vi "数据收集.vi"(8 "error in (no error)":errorcluster caption="错误输入（无错误）", 9 "DB5000.X":T1, 10 "Value":dbl format="%_3g", 11 "数组in":dbl[][](array[numeric])) -> (0 "error out":errorcluster caption="错误输出", 1 "添加的数组":dbl[](array[numeric]), 2 "连接的字符串":string, 3 "数组out":dbl[][](array[numeric]))   [LabVIEW 2017]
uses:
  <vilib>/Utility/file.llb/Write Delimited Spreadsheet (DBL).vi
panel:
  out "元素":bool
  out "F-格式字符串":string[](array[string])
  out "添加的数组 19":dbl[](array[numeric])
  out "MAX位置2":dbl format="%#_3g"
  out "添加的数组 20":dbl[](array[numeric])
  out "MAX位置1":dbl format="%#_3g"
  out "添加的数组 17":dbl[](array[numeric])
  out "MAX位置3":dbl format="%#_3g"
  out "添加的数组 18":dbl[](array[numeric])
  out "MAX位置18":dbl format="%#_3g"
  out "添加的数组 21":dbl[](array[numeric])
  out "MAX位置19":dbl format="%#_3g"
  out "添加的数组 14":dbl[](array[numeric])
  out "MAX位置17":dbl format="%#_3g"
  out "添加的数组 15":dbl[](array[numeric])
  out "MAX位置16":dbl format="%#_3g"
  out "添加的数组 16":dbl[](array[numeric])
  out "MAX位置15":dbl format="%#_3g"
  out "添加的数组 11":dbl[](array[numeric])
  out "MAX位置14":dbl format="%#_3g"
  out "添加的数组 12":dbl[](array[numeric])
  out "MAX位置13":dbl format="%#_3g"
  out "添加的数组 10":dbl[](array[numeric])
  out "MAX位置12":dbl format="%#_3g"
  out "添加的数组 9":dbl[](array[numeric])
  out "MAX位置11":dbl format="%#_3g"
  out "添加的数组 8":dbl[](array[numeric])
  out "MAX位置10":dbl format="%#_3g"
  out "添加的数组 7":dbl[](array[numeric])
  out "MAX位置9":dbl format="%#_3g"
  out "添加的数组 6":dbl[](array[numeric])
  out "MAX位置8":dbl format="%#_3g"
  out "添加的数组 5":dbl[](array[numeric])
  out "MAX位置7":dbl format="%#_3g"
  out "添加的数组 4":dbl[](array[numeric])
  out "MAX位置6":dbl format="%#_3g"
  out "添加的数组 3":dbl[](array[numeric])
  out "MAX位置5":dbl format="%#_3g"
  out "添加的数组 2":dbl[](array[numeric])
  out "MAX位置4":dbl format="%#_3g"
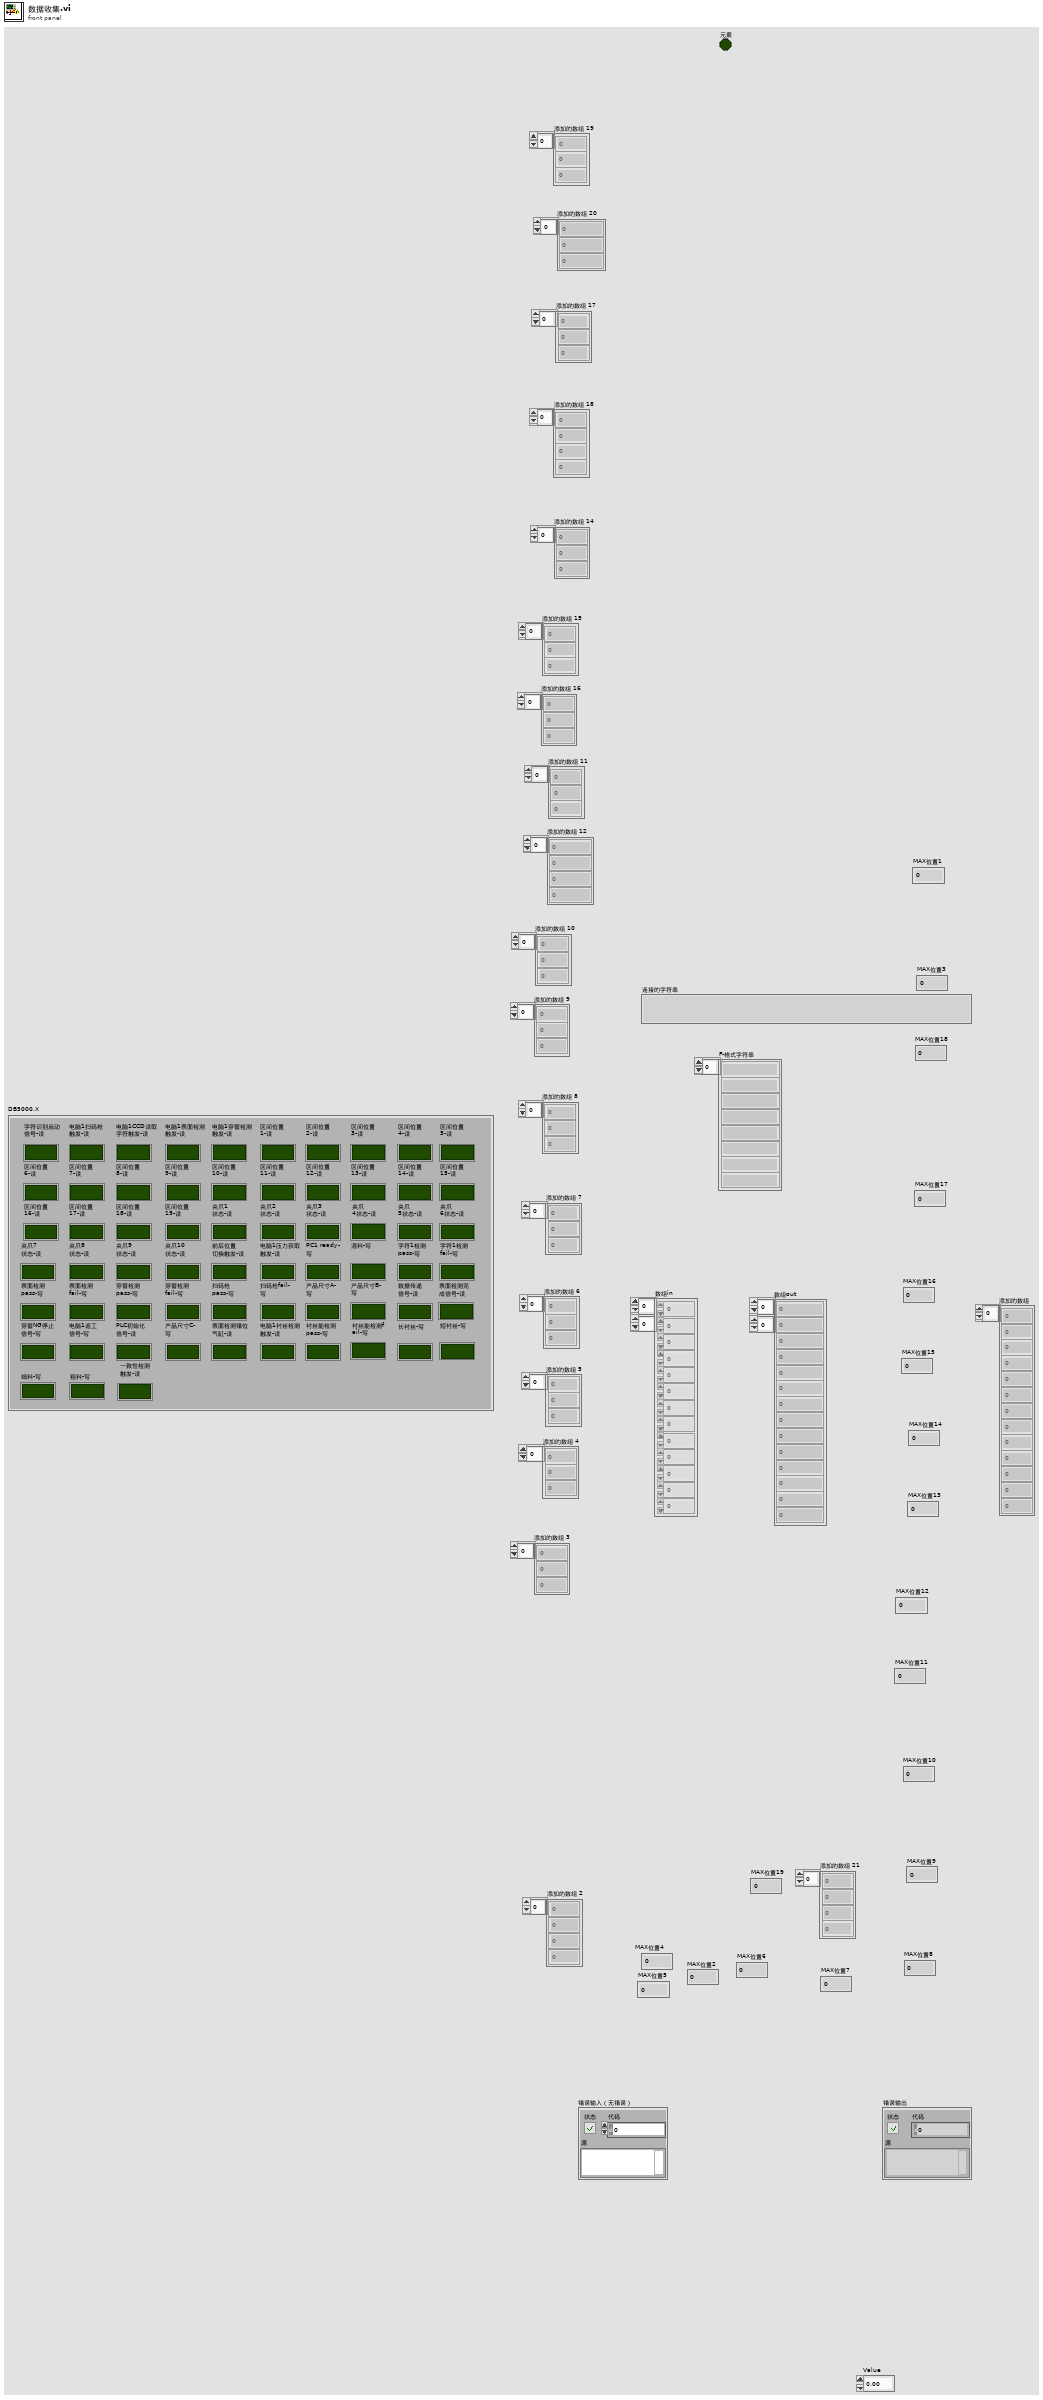
[diagram p1: front panel]
types:
  T1 = cluster{"字符识别启动\n信号-读":bool, "电脑1扫码枪\n触发-读":bool, "电脑1CCD读取\n字符触发-读":bool, "电脑1表面检测\n触发-读":bool, "电脑1穿管检测\n触发-读":bool, "区间位置\n1-读":bool, "区间位置\n2-读":bool, "区间位置\n3-读":bool, "区间位置\n4-读":bool, "区间位置\n5-读":bool, "区间位置\n6-读":bool, "区间位置\n7-读":bool, "区间位置\n8-读":bool, "区间位置\n9-读":bool, "区间位置\n10-读":bool, "区间位置\n11-读":bool, "区间位置\n12-读":bool, "区间位置\n13-读":bool, "区间位置\n14-读":bool, "区间位置\n15-读":bool, "区间位置\n16-读":bool, "区间位置\n17-读":bool, "区间位置\n18-读":bool, "区间位置\n19-读":bool, "夹爪1\n状态-读":bool, "夹爪2\n状态-读":bool, "夹爪3\n状态-读":bool, "夹爪\n4状态-读":bool, "夹爪\n5状态-读":bool, "夹爪\n6状态-读":bool, "夹爪7\n状态-读":bool, "夹爪8\n状态-读":bool, "夹爪9\n状态-读":bool, "夹爪10\n状态-读":bool, "前后位置\n切换触发-读":bool, "电脑1压力获取\n触发-读":bool, "PC1 ready-\n写 ":bool, "混料-写\n":bool, "字符1检测\npass-写":bool, "字符1检测\nfail-写":bool, "表面检测\npass-写":bool, "表面检测\nfail-写":bool, "穿管检测\npass-写":bool, "穿管检测\nfail-写":bool, "扫码枪\npass-写":bool, "扫码枪fail-\n写":bool, "产品尺寸A-\n写":bool, "产品尺寸B-\n写":bool, "数据传递\n信号-读":bool, "表面检测完\n成信号-读":bool, "穿管NG停止\n信号-写":bool, "电脑1返工\n信号-写":bool, "PLC初始化\n信号-读":bool, "产品尺寸C-\n写":bool, "表面检测错位\n气缸-读":bool, "电脑1衬丝检测\n触发-读":bool, "衬丝能检测\npass-写":bool, "衬丝能检测f\nail-写":bool, "长衬丝-写\n":bool, "短衬丝-写\n":bool, "细料-写":bool, "粗料-写":bool, "一致性检测\n触发-读":bool}
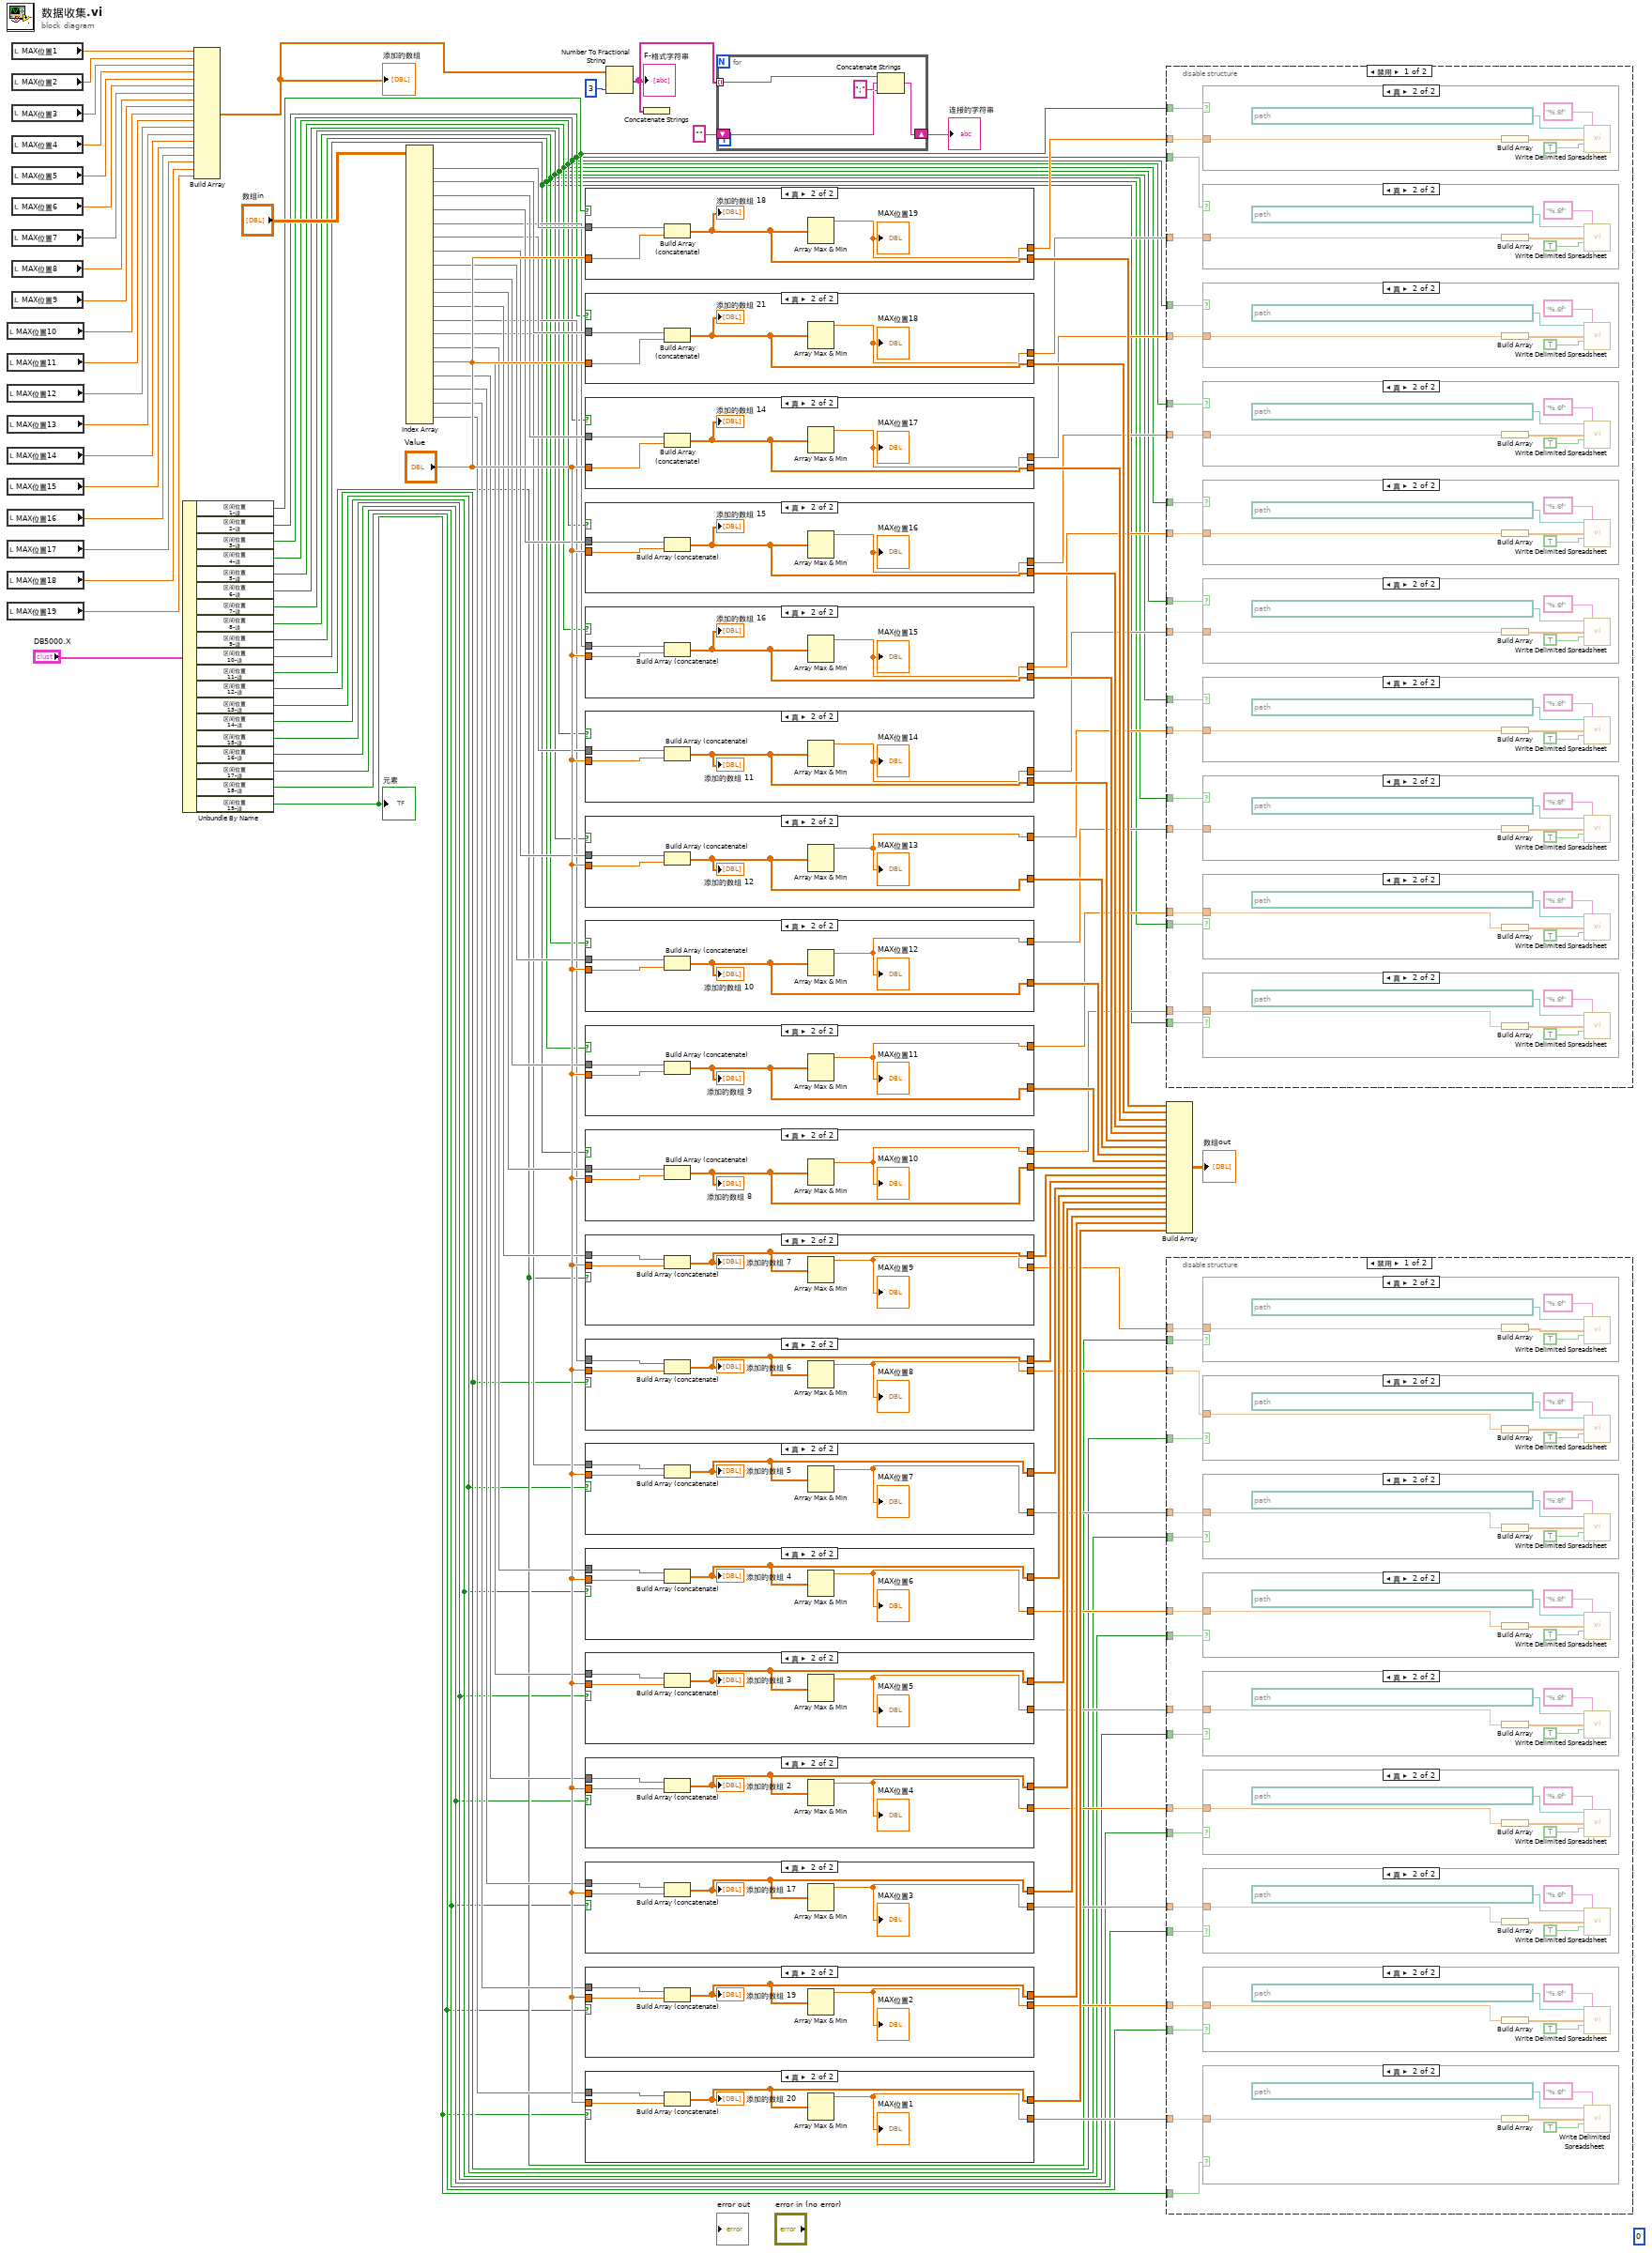
[diagram p0: block diagram]
diagram:
  (unwired) 0 ("索引")
  n1 = local read "MAX位置10"() -> (w97:dbl)
  n2 = local read "MAX位置11"() -> (w96:dbl)
  n3 = local read "MAX位置12"() -> (w95:dbl)
  n4 = local read "MAX位置13"() -> (w94:dbl)
  n5 = local read "MAX位置14"() -> (w93:dbl)
  n6 = local read "MAX位置15"() -> (w92:dbl)
  n7 = local read "MAX位置16"() -> (w91:dbl)
  n8 = local read "MAX位置17"() -> (w90:dbl)
  n9 = local read "MAX位置18"() -> (w89:dbl)
  n10 = local read "MAX位置19"() -> (w88:dbl)
  n11 = local read "MAX位置1"() -> (w47:dbl)
  n12 = local read "MAX位置2"() -> (w46:dbl)
  n13 = local read "MAX位置3"() -> (w45:dbl)
  n14 = local read "MAX位置4"() -> (w103:dbl)
  n15 = local read "MAX位置5"() -> (w102:dbl)
  n16 = local read "MAX位置6"() -> (w101:dbl)
  n17 = local read "MAX位置7"() -> (w100:dbl)
  n18 = local read "MAX位置8"() -> (w99:dbl)
  n19 = local read "MAX位置9"() -> (w98:dbl)
  n20 = Unbundle By Name("DB5000.X") -> ("区间位置\n1-读"=w19:bool, "区间位置\n2-读"=w18:bool, "区间位置\n3-读"=w17:bool, "区间位置\n4-读"=w16:bool, "区间位置\n5-读"=w15:bool, "区间位置\n6-读"=w14:bool, "区间位置\n7-读"=w13:bool, "区间位置\n8-读"=w12:bool, "区间位置\n9-读"=w11:bool, "区间位置\n10-读"=w10:bool, "区间位置\n11-读"=w9:bool, "区间位置\n12-读"=w8:bool, "区间位置\n13-读"=w7:bool, "区间位置\n14-读"=w6:bool, "区间位置\n15-读"=w5:bool, "区间位置\n16-读"=w4:bool, "区间位置\n17-读"=w3:bool, "区间位置\n18-读"=w2:bool, "区间位置\n19-读"=w1:bool)
  "元素" <- w1
  n21 = Build Array(w47, w46, w45, w103, w102, w101, w100, w99, w98, w97, w96, w95, w94, w93, w92, w91, w90, w89, w88) -> (w44:dbl[])
  "添加的数组" <- w44
  n22 = Index Array(array="数组in") -> (element #1=w86:dbl[], element #2=w85:dbl[], element #3=w84:dbl[], element #4=w83:dbl[], element #5=w82:dbl[], element #6=w81:dbl[], element #7=w80:dbl[], element #8=w79:dbl[], element #9=w78:dbl[], element #10=w77:dbl[], element #11=w76:dbl[], element #12=w48:dbl[], element #13=w75:dbl[], element #14=w74:dbl[], element #15=w73:dbl[], element #16=w72:dbl[], element #17=w71:dbl[], element #18=w70:dbl[], element #19=w69:dbl[])  [unwired: 38 in]
  n23 = case shown="真" w19 {
    tunnel: [dbl[] [] ("添加的数组") w108] -> w68
    tunnel: "Value" -> [_ w109]
    tunnel: w86 -> [_ w107]
    tunnel: [_ w106] -> w39
    frame False {
    }
    frame True {
      n24 = Build Array (concatenate)(w107, w109) -> (w108:dbl[])
      "添加的数组 18" <- w108
      n25 = Array Max & Min(array=w108) -> (max value=w106:dbl)  [unwired: 3 out]
      "MAX位置19" <- w106
    }
  }
  n26 = case shown="真" w18 {
    tunnel: [dbl[] [] ("添加的数组") w113] -> w67
    tunnel: "Value" -> [_ w114]
    tunnel: w85 -> [_ w112]
    tunnel: [_ w111] -> w38
    frame False {
    }
    frame True {
      n27 = Build Array (concatenate)(w112, w114) -> (w113:dbl[])
      "添加的数组 21" <- w113
      n28 = Array Max & Min(array=w113) -> (max value=w111:dbl)  [unwired: 3 out]
      "MAX位置18" <- w111
    }
  }
  n29 = case shown="真" w17 {
    tunnel: [dbl[] [] ("添加的数组") w118] -> w66
    tunnel: "Value" -> [_ w119]
    tunnel: w84 -> [_ w117]
    tunnel: [_ w116] -> w37
    frame False {
    }
    frame True {
      n30 = Build Array (concatenate)(w117, w119) -> (w118:dbl[])
      "添加的数组 14" <- w118
      n31 = Array Max & Min(array=w118) -> (max value=w116:dbl)  [unwired: 3 out]
      "MAX位置17" <- w116
    }
  }
  n32 = case shown="真" w16 {
    tunnel: [dbl[] [] ("添加的数组") w123] -> w65
    tunnel: "Value" -> [_ w124]
    tunnel: w83 -> [_ w122]
    tunnel: [_ w121] -> w36
    frame False {
    }
    frame True {
      n33 = Build Array (concatenate)(w122, w124) -> (w123:dbl[])
      "添加的数组 15" <- w123
      n34 = Array Max & Min(array=w123) -> (max value=w121:dbl)  [unwired: 3 out]
      "MAX位置16" <- w121
    }
  }
  n35 = case shown="真" w15 {
    tunnel: [dbl[] [] ("添加的数组") w128] -> w64
    tunnel: "Value" -> [_ w129]
    tunnel: w82 -> [_ w127]
    tunnel: [_ w126] -> w35
    frame False {
    }
    frame True {
      n36 = Build Array (concatenate)(w127, w129) -> (w128:dbl[])
      "添加的数组 16" <- w128
      n37 = Array Max & Min(array=w128) -> (max value=w126:dbl)  [unwired: 3 out]
      "MAX位置15" <- w126
    }
  }
  n38 = case shown="真" w14 {
    tunnel: [dbl[] [] ("添加的数组") w133] -> w63
    tunnel: "Value" -> [_ w134]
    tunnel: w81 -> [_ w132]
    tunnel: [_ w131] -> w34
    frame False {
    }
    frame True {
      n39 = Build Array (concatenate)(w132, w134) -> (w133:dbl[])
      "添加的数组 11" <- w133
      n40 = Array Max & Min(array=w133) -> (max value=w131:dbl)  [unwired: 3 out]
      "MAX位置14" <- w131
    }
  }
  n41 = case shown="真" w13 {
    tunnel: [dbl[] [] ("添加的数组") w138] -> w62
    tunnel: "Value" -> [_ w139]
    tunnel: w80 -> [_ w137]
    tunnel: [_ w136] -> w21
    frame False {
    }
    frame True {
      n42 = Build Array (concatenate)(w137, w139) -> (w138:dbl[])
      "添加的数组 12" <- w138
      n43 = Array Max & Min(array=w138) -> (max value=w136:dbl)  [unwired: 3 out]
      "MAX位置13" <- w136
    }
  }
  n44 = case shown="真" w12 {
    tunnel: [dbl[] [] ("添加的数组") w143] -> w61
    tunnel: "Value" -> [_ w144]
    tunnel: w79 -> [_ w142]
    tunnel: [_ w141] -> w22
    frame False {
    }
    frame True {
      n45 = Build Array (concatenate)(w142, w144) -> (w143:dbl[])
      "添加的数组 10" <- w143
      n46 = Array Max & Min(array=w143) -> (max value=w141:dbl)  [unwired: 3 out]
      "MAX位置12" <- w141
    }
  }
  n47 = case shown="真" w11 {
    tunnel: [dbl[] [] ("添加的数组") w148] -> w60
    tunnel: "Value" -> [_ w149]
    tunnel: w78 -> [_ w147]
    tunnel: [_ w146] -> w23
    frame False {
    }
    frame True {
      n48 = Build Array (concatenate)(w147, w149) -> (w148:dbl[])
      "添加的数组 9" <- w148
      n49 = Array Max & Min(array=w148) -> (max value=w146:dbl)  [unwired: 3 out]
      "MAX位置11" <- w146
    }
  }
  n50 = case shown="真" w10 {
    tunnel: [dbl[] [] ("添加的数组") w153] -> w59
    tunnel: "Value" -> [_ w154]
    tunnel: w77 -> [_ w152]
    tunnel: [_ w151] -> w24
    frame False {
    }
    frame True {
      n51 = Build Array (concatenate)(w152, w154) -> (w153:dbl[])
      "添加的数组 8" <- w153
      n52 = Array Max & Min(array=w153) -> (max value=w151:dbl)  [unwired: 3 out]
      "MAX位置10" <- w151
    }
  }
  n53 = case shown="真" w9 {
    tunnel: [dbl[] [] ("添加的数组") w158] -> w58
    tunnel: "Value" -> [_ w159]
    tunnel: w76 -> [_ w157]
    tunnel: [_ w156] -> w25
    frame False {
    }
    frame True {
      n54 = Build Array (concatenate)(w157, w159) -> (w158:dbl[])
      "添加的数组 7" <- w158
      n55 = Array Max & Min(array=w158) -> (max value=w156:dbl)  [unwired: 3 out]
      "MAX位置9" <- w156
    }
  }
  n56 = case shown="真" w8 {
    tunnel: [dbl[] [] ("添加的数组") w163] -> w57
    tunnel: "Value" -> [_ w164]
    tunnel: w48 -> [_ w162]
    tunnel: [_ w161] -> w26
    frame False {
    }
    frame True {
      n57 = Build Array (concatenate)(w162, w164) -> (w163:dbl[])
      "添加的数组 6" <- w163
      n58 = Array Max & Min(array=w163) -> (max value=w161:dbl)  [unwired: 3 out]
      "MAX位置8" <- w161
    }
  }
  n59 = case shown="真" w7 {
    tunnel: [dbl[] [] ("添加的数组") w168] -> w56
    tunnel: "Value" -> [_ w169]
    tunnel: w75 -> [_ w167]
    tunnel: [_ w166] -> w27
    frame False {
    }
    frame True {
      n60 = Build Array (concatenate)(w167, w169) -> (w168:dbl[])
      "添加的数组 5" <- w168
      n61 = Array Max & Min(array=w168) -> (max value=w166:dbl)  [unwired: 3 out]
      "MAX位置7" <- w166
    }
  }
  n62 = case shown="真" w6 {
    tunnel: [dbl[] [] ("添加的数组") w173] -> w55
    tunnel: "Value" -> [_ w174]
    tunnel: w74 -> [_ w172]
    tunnel: [_ w171] -> w28
    frame False {
    }
    frame True {
      n63 = Build Array (concatenate)(w172, w174) -> (w173:dbl[])
      "添加的数组 4" <- w173
      n64 = Array Max & Min(array=w173) -> (max value=w171:dbl)  [unwired: 3 out]
      "MAX位置6" <- w171
    }
  }
  n65 = case shown="真" w5 {
    tunnel: [dbl[] [] ("添加的数组") w178] -> w54
    tunnel: "Value" -> [_ w179]
    tunnel: w73 -> [_ w177]
    tunnel: [_ w176] -> w29
    frame False {
    }
    frame True {
      n66 = Build Array (concatenate)(w177, w179) -> (w178:dbl[])
      "添加的数组 3" <- w178
      n67 = Array Max & Min(array=w178) -> (max value=w176:dbl)  [unwired: 3 out]
      "MAX位置5" <- w176
    }
  }
  n68 = case shown="真" w4 {
    tunnel: [dbl[] [] ("添加的数组") w183] -> w53
    tunnel: "Value" -> [_ w184]
    tunnel: w72 -> [_ w182]
    tunnel: [_ w181] -> w30
    frame False {
    }
    frame True {
      n69 = Build Array (concatenate)(w182, w184) -> (w183:dbl[])
      "添加的数组 2" <- w183
      n70 = Array Max & Min(array=w183) -> (max value=w181:dbl)  [unwired: 3 out]
      "MAX位置4" <- w181
    }
  }
  n71 = case shown="真" w3 {
    tunnel: [dbl[] [] ("添加的数组") w188] -> w52
    tunnel: "Value" -> [_ w189]
    tunnel: w71 -> [_ w187]
    tunnel: [_ w186] -> w31
    frame False {
    }
    frame True {
      n72 = Build Array (concatenate)(w187, w189) -> (w188:dbl[])
      "添加的数组 17" <- w188
      n73 = Array Max & Min(array=w188) -> (max value=w186:dbl)  [unwired: 3 out]
      "MAX位置3" <- w186
    }
  }
  n74 = case shown="真" w2 {
    tunnel: [dbl[] [] ("添加的数组") w193] -> w51
    tunnel: "Value" -> [_ w194]
    tunnel: w70 -> [_ w192]
    tunnel: [_ w191] -> w32
    frame False {
    }
    frame True {
      n75 = Build Array (concatenate)(w192, w194) -> (w193:dbl[])
      "添加的数组 19" <- w193
      n76 = Array Max & Min(array=w193) -> (max value=w191:dbl)  [unwired: 3 out]
      "MAX位置2" <- w191
    }
  }
  n77 = case shown="真" w1 {
    tunnel: [dbl[] [] ("添加的数组") w198] -> w50
    tunnel: "Value" -> [_ w199]
    tunnel: w69 -> [_ w197]
    tunnel: [_ w196] -> w33
    frame False {
    }
    frame True {
      n78 = Build Array (concatenate)(w197, w199) -> (w198:dbl[])
      "添加的数组 20" <- w198
      n79 = Array Max & Min(array=w198) -> (max value=w196:dbl)  [unwired: 3 out]
      "MAX位置1" <- w196
    }
  }
  n80 = Number To Fractional String(number=w44, precision (6)=i16 3 ("精度(6)")) -> (F-format string=w42:string[])  [unwired: 2 in]
  "F-格式字符串" <- w42
  n81 = Concatenate Strings(w42) -> ()  [unwired: 1 out]
  n82 = for {
    tunnel: w42 -> [w203] mode=indexing
    shift-right: [w200] -> w40
    shift-left: "" -> [w201]
    n83 = Concatenate Strings(w203, ";" ("字符串"), w201) -> (w200:string)
  }
  "连接的字符串" <- w40
  n84 = disable-structure shown="禁用" {
    disable-tunnel: w39 -> [w223 _]
    disable-tunnel: w38 -> [w222 _]
    disable-tunnel: w37 -> [w221 _]
    disable-tunnel: w36 -> [w220 _]
    disable-tunnel: w35 -> [w219 _]
    disable-tunnel: w34 -> [w218 _]
    disable-tunnel: w24 -> [w217 _]
    disable-tunnel: w23 -> [w216 _]
    disable-tunnel: w22 -> [w215 _]
    disable-tunnel: w21 -> [w214 _]
    disable-tunnel: w19 -> [w213 _]
    disable-tunnel: w18 -> [w212 _]
    disable-tunnel: w17 -> [w211 _]
    disable-tunnel: w16 -> [w210 _]
    disable-tunnel: w15 -> [w209 _]
    disable-tunnel: w14 -> [w208 _]
    disable-tunnel: w13 -> [w207 _]
    disable-tunnel: w12 -> [w206 _]
    disable-tunnel: w11 -> [w205 _]
    disable-tunnel: w10 -> [w204 _]
    frame Disabled {
      n85 = case shown="真" w213 {
        tunnel: w223 -> [_ w264]
        frame False {
        }
        frame True {
          n86 = Build Array(w264) -> (w265:dbl[])
          n87 = call-poly <vilib>:"Write Delimited Spreadsheet.vi"("file path (dialog if empty)"=path "C:/Users/Administrator/Desktop/新建文件夹/新建文本文档 - 副本 (19).txt", "format (%.3f)"="%.6f", "1D data"=w265, "append to file? (new file:F)"=TRUE) -> ()  [unwired: 10 in, 2 out]
        }
      }
      n88 = case shown="真" w212 {
        tunnel: w222 -> [_ w259]
        frame False {
        }
        frame True {
          n89 = Build Array(w259) -> (w260:dbl[])
          n90 = call-poly <vilib>:"Write Delimited Spreadsheet.vi"("file path (dialog if empty)"=path "C:/Users/Administrator/Desktop/新建文件夹/新建文本文档 - 副本 (18).txt", "format (%.3f)"="%.6f", "1D data"=w260, "append to file? (new file:F)"=TRUE) -> ()  [unwired: 10 in, 2 out]
        }
      }
      n91 = case shown="真" w211 {
        tunnel: w221 -> [_ w254]
        frame False {
        }
        frame True {
          n92 = Build Array(w254) -> (w255:dbl[])
          n93 = call-poly <vilib>:"Write Delimited Spreadsheet.vi"("file path (dialog if empty)"=path "C:/Users/Administrator/Desktop/新建文件夹/新建文本文档 - 副本 (17).txt", "format (%.3f)"="%.6f", "1D data"=w255, "append to file? (new file:F)"=TRUE) -> ()  [unwired: 10 in, 2 out]
        }
      }
      n94 = case shown="真" w210 {
        tunnel: w220 -> [_ w249]
        frame False {
        }
        frame True {
          n95 = Build Array(w249) -> (w250:dbl[])
          n96 = call-poly <vilib>:"Write Delimited Spreadsheet.vi"("file path (dialog if empty)"=path "C:/Users/Administrator/Desktop/新建文件夹/新建文本文档 - 副本 (16).txt", "format (%.3f)"="%.6f", "1D data"=w250, "append to file? (new file:F)"=TRUE) -> ()  [unwired: 10 in, 2 out]
        }
      }
      n97 = case shown="真" w209 {
        tunnel: w219 -> [_ w244]
        frame False {
        }
        frame True {
          n98 = Build Array(w244) -> (w245:dbl[])
          n99 = call-poly <vilib>:"Write Delimited Spreadsheet.vi"("file path (dialog if empty)"=path "C:/Users/Administrator/Desktop/新建文件夹/新建文本文档 - 副本 (15).txt", "format (%.3f)"="%.6f", "1D data"=w245, "append to file? (new file:F)"=TRUE) -> ()  [unwired: 10 in, 2 out]
        }
      }
      n100 = case shown="真" w208 {
        tunnel: w218 -> [_ w239]
        frame False {
        }
        frame True {
          n101 = Build Array(w239) -> (w240:dbl[])
          n102 = call-poly <vilib>:"Write Delimited Spreadsheet.vi"("file path (dialog if empty)"=path "C:/Users/Administrator/Desktop/新建文件夹/新建文本文档 - 副本 (14).txt", "format (%.3f)"="%.6f", "1D data"=w240, "append to file? (new file:F)"=TRUE) -> ()  [unwired: 10 in, 2 out]
        }
      }
      n103 = case shown="真" w207 {
        tunnel: w214 -> [_ w269]
        frame False {
        }
        frame True {
          n104 = Build Array(w269) -> (w270:dbl[])
          n105 = call-poly <vilib>:"Write Delimited Spreadsheet.vi"("file path (dialog if empty)"=path "C:/Users/Administrator/Desktop/新建文件夹/新建文本文档 - 副本 (13).txt", "format (%.3f)"="%.6f", "1D data"=w270, "append to file? (new file:F)"=TRUE) -> ()  [unwired: 10 in, 2 out]
        }
      }
      n106 = case shown="真" w206 {
        tunnel: w215 -> [_ w234]
        frame False {
        }
        frame True {
          n107 = Build Array(w234) -> (w235:dbl[])
          n108 = call-poly <vilib>:"Write Delimited Spreadsheet.vi"("file path (dialog if empty)"=path "C:/Users/Administrator/Desktop/新建文件夹/新建文本文档 - 副本 (12).txt", "format (%.3f)"="%.6f", "1D data"=w235, "append to file? (new file:F)"=TRUE) -> ()  [unwired: 10 in, 2 out]
        }
      }
      n109 = case shown="真" w205 {
        tunnel: w216 -> [_ w229]
        frame False {
        }
        frame True {
          n110 = Build Array(w229) -> (w230:dbl[])
          n111 = call-poly <vilib>:"Write Delimited Spreadsheet.vi"("file path (dialog if empty)"=path "C:/Users/Administrator/Desktop/新建文件夹/新建文本文档 - 副本 (11).txt", "format (%.3f)"="%.6f", "1D data"=w230, "append to file? (new file:F)"=TRUE) -> ()  [unwired: 10 in, 2 out]
        }
      }
      n112 = case shown="真" w204 {
        tunnel: w217 -> [_ w224]
        frame False {
        }
        frame True {
          n113 = Build Array(w224) -> (w225:dbl[])
          n114 = call-poly <vilib>:"Write Delimited Spreadsheet.vi"("file path (dialog if empty)"=path "C:/Users/Administrator/Desktop/新建文件夹/新建文本文档 - 副本 (10).txt", "format (%.3f)"="%.6f", "1D data"=w225, "append to file? (new file:F)"=TRUE) -> ()  [unwired: 10 in, 2 out]
        }
      }
    }
    frame Enabled {
    }
  }
  n115 = Build Array(w68, w67, w66, w65, w64, w63, w62, w61, w60, w59, w58, w57, w56, w55, w54, w53, w52, w51, w50) -> (→"数组out":dbl[][])
  n116 = disable-structure shown="禁用" {
    disable-tunnel: w33 -> [w291 _]
    disable-tunnel: w32 -> [w290 _]
    disable-tunnel: w31 -> [w289 _]
    disable-tunnel: w30 -> [w288 _]
    disable-tunnel: w29 -> [w287 _]
    disable-tunnel: w28 -> [w286 _]
    disable-tunnel: w27 -> [w285 _]
    disable-tunnel: w26 -> [w284 _]
    disable-tunnel: w25 -> [w283 _]
    disable-tunnel: w9 -> [w282 _]
    disable-tunnel: w8 -> [w281 _]
    disable-tunnel: w7 -> [w280 _]
    disable-tunnel: w6 -> [w279 _]
    disable-tunnel: w5 -> [w278 _]
    disable-tunnel: w4 -> [w277 _]
    disable-tunnel: w3 -> [w276 _]
    disable-tunnel: w2 -> [w275 _]
    disable-tunnel: w1 -> [w274 _]
    frame Disabled {
      n117 = case shown="真" w282 {
        tunnel: w283 -> [_ w317]
        frame False {
        }
        frame True {
          n118 = Build Array(w317) -> (w318:dbl[])
          n119 = call-poly <vilib>:"Write Delimited Spreadsheet.vi"("file path (dialog if empty)"=path "C:/Users/Administrator/Desktop/新建文件夹/新建文本文档 - 副本 (9).txt", "format (%.3f)"="%.6f", "1D data"=w318, "append to file? (new file:F)"=TRUE) -> ()  [unwired: 10 in, 2 out]
        }
      }
      n120 = case shown="真" w281 {
        tunnel: w284 -> [_ w312]
        frame False {
        }
        frame True {
          n121 = Build Array(w312) -> (w313:dbl[])
          n122 = call-poly <vilib>:"Write Delimited Spreadsheet.vi"("file path (dialog if empty)"=path "C:/Users/Administrator/Desktop/新建文件夹/新建文本文档 - 副本 (8).txt", "format (%.3f)"="%.6f", "1D data"=w313, "append to file? (new file:F)"=TRUE) -> ()  [unwired: 10 in, 2 out]
        }
      }
      n123 = case shown="真" w280 {
        tunnel: w285 -> [_ w332]
        frame False {
        }
        frame True {
          n124 = Build Array(w332) -> (w333:dbl[])
          n125 = call-poly <vilib>:"Write Delimited Spreadsheet.vi"("file path (dialog if empty)"=path "C:/Users/Administrator/Desktop/新建文件夹/新建文本文档 - 副本 (7).txt", "format (%.3f)"="%.6f", "1D data"=w333, "append to file? (new file:F)"=TRUE) -> ()  [unwired: 10 in, 2 out]
        }
      }
      n126 = case shown="真" w279 {
        tunnel: w286 -> [_ w327]
        frame False {
        }
        frame True {
          n127 = Build Array(w327) -> (w328:dbl[])
          n128 = call-poly <vilib>:"Write Delimited Spreadsheet.vi"("file path (dialog if empty)"=path "C:/Users/Administrator/Desktop/新建文件夹/新建文本文档 - 副本 (6).txt", "format (%.3f)"="%.6f", "1D data"=w328, "append to file? (new file:F)"=TRUE) -> ()  [unwired: 10 in, 2 out]
        }
      }
      n129 = case shown="真" w278 {
        tunnel: w287 -> [_ w307]
        frame False {
        }
        frame True {
          n130 = Build Array(w307) -> (w308:dbl[])
          n131 = call-poly <vilib>:"Write Delimited Spreadsheet.vi"("file path (dialog if empty)"=path "C:/Users/Administrator/Desktop/新建文件夹/新建文本文档 - 副本 (5).txt", "format (%.3f)"="%.6f", "1D data"=w308, "append to file? (new file:F)"=TRUE) -> ()  [unwired: 10 in, 2 out]
        }
      }
      n132 = case shown="真" w277 {
        tunnel: w288 -> [_ w302]
        frame False {
        }
        frame True {
          n133 = Build Array(w302) -> (w303:dbl[])
          n134 = call-poly <vilib>:"Write Delimited Spreadsheet.vi"("file path (dialog if empty)"=path "C:/Users/Administrator/Desktop/新建文件夹/新建文本文档 - 副本 (4).txt", "format (%.3f)"="%.6f", "1D data"=w303, "append to file? (new file:F)"=TRUE) -> ()  [unwired: 10 in, 2 out]
        }
      }
      n135 = case shown="真" w276 {
        tunnel: w289 -> [_ w297]
        frame False {
        }
        frame True {
          n136 = Build Array(w297) -> (w298:dbl[])
          n137 = call-poly <vilib>:"Write Delimited Spreadsheet.vi"("file path (dialog if empty)"=path "C:/Users/Administrator/Desktop/新建文件夹/新建文本文档 - 副本 (3).txt", "format (%.3f)"="%.6f", "1D data"=w298, "append to file? (new file:F)"=TRUE) -> ()  [unwired: 10 in, 2 out]
        }
      }
      n138 = case shown="真" w275 {
        tunnel: w290 -> [_ w322]
        frame False {
        }
        frame True {
          n139 = Build Array(w322) -> (w323:dbl[])
          n140 = call-poly <vilib>:"Write Delimited Spreadsheet.vi"("file path (dialog if empty)"=path "C:/Users/Administrator/Desktop/新建文件夹/新建文本文档 - 副本 (2).txt", "format (%.3f)"="%.6f", "1D data"=w323, "append to file? (new file:F)"=TRUE) -> ()  [unwired: 10 in, 2 out]
        }
      }
      n141 = case shown="真" w274 {
        tunnel: w291 -> [_ w292]
        frame False {
        }
        frame True {
          n142 = Build Array(w292) -> (w293:dbl[])
          n143 = call-poly <vilib>:"Write Delimited Spreadsheet.vi"("file path (dialog if empty)"=path "C:/Users/Administrator/Desktop/新建文件夹/新建文本文档 - 副本.txt", "format (%.3f)"="%.6f", "1D data"=w293, "append to file? (new file:F)"=TRUE) -> ()  [unwired: 10 in, 2 out]
        }
      }
    }
    frame Enabled {
    }
  }
